vi "RSZVB Query Measurement Parameters.vi"(8 "error in (no error)":errorcluster {"code" format="%.0x"}, 9 "Trace Name (Trc1)":string="Trc1", 10 "Channel (1)":i32=1, 11 "VISA session":refnum<visa-resource-name>) -> (0 "error out":errorcluster {"code" format="%.0x"}, 2 "Parameters":string, 3 "dup VISA session":refnum<visa-resource-name>)   [LabVIEW 2011]
doc: "This VI queries a measurement parameter of an existing trace. \n\nRemote-control command(s):\nCALCulate<Ch>:PARameter:MEASure? '<string>'"
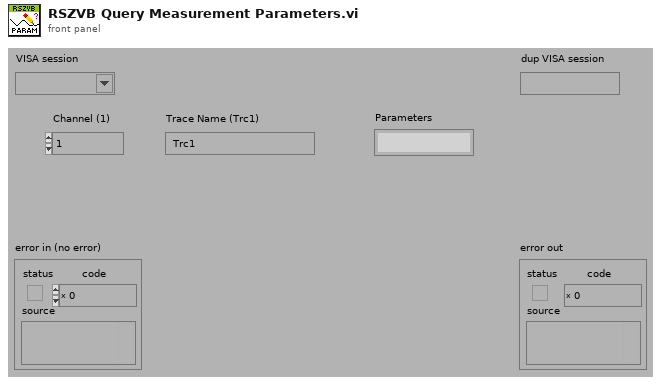
[diagram p1: front panel]
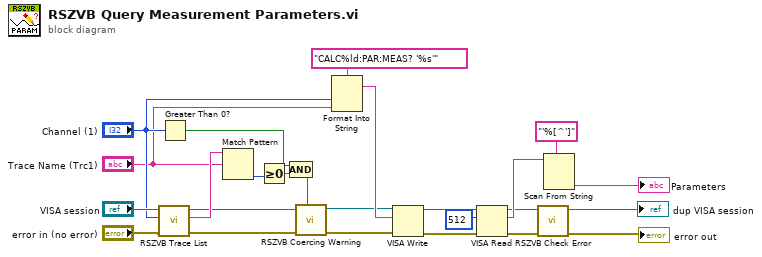
[diagram p0: block diagram]
diagram:
  n1 = call "RSZVB Trace List.vi"("error in (no error)"="error in (no error)", "Channel (1)"="Channel (1)", "VISA session"="VISA session") -> ("error out"=w13:errorcluster, "Catalog"=w20:string, "dup VISA session"=w14:refnum<visa-resource-name>)  [unwired: 6 in]
  n2 = Greater Than 0?(x="Channel (1)") -> (x > 0?=w16:bool)
  n3 = Match Pattern(string=w20, regular expression="Trace Name (Trc1)") -> (offset past match=w19:i32)  [unwired: 1 in, 3 out]
  n4 = Greater Or Equal To 0?(x=w19) -> (x >= 0?=w15:bool)
  n5 = Compound Arithmetic op=AND(w16, w15) -> (w24:bool)
  n6 = call "RSZVB Coercing Warning.vi"("In Range?"=w24, "error in (no error)"=w13, "VISA session"=w14) -> ("error out"=w9:errorcluster, "dup VISA session"=w10:refnum<visa-resource-name>)  [unwired: 7 in]
  n7 = Format Into String(format string="CALC%ld:PAR:MEAS? '%s'", "Channel (1)", "Trace Name (Trc1)") -> (resulting string=w23:string)  [unwired: 2 in, 1 out]
  n8 = VISA Write(VISA resource name=w10, write buffer=w23, error in (no error)=w9) -> (VISA resource name out=w5:refnum<visa-resource-name>, error out=w4:errorcluster)  [unwired: 1 out]
  n9 = VISA Read(VISA resource name=w5, byte count=u32 512 ("byte count (0)"), error in (no error)=w4) -> (VISA resource name out=w2:refnum<visa-resource-name>, read buffer=w6:string, error out=w1:errorcluster)  [unwired: 1 out]
  n10 = call "RSZVB Check Error.vi"("error in (no error)"=w1, "VISA session"=w2) -> ("error out"=→"error out":errorcluster, "dup VISA session"=→"dup VISA session":refnum<visa-resource-name>)  [unwired: 8 in]
  n11 = Scan From String(format string="'%[^']", input string=w6) -> (output 1=→"Parameters":string)  [unwired: 3 in, 3 out]
